vi "CleanUp.vi"(0 "object in":refnum<class "AD2andExtAWG.lvclass">, 5 "error in (no error)":errorcluster) -> (14 "object out":refnum<class "AD2andExtAWG.lvclass">, 19 "error out":errorcluster)   [LabVIEW 2019, in "AD2andExtAWG.lvclass"]
uses:
  AD2andExtAWG.lvclass
  AD2_SDK_class/AD2_SDK.lvclass
  AFG3022B_class/AFG3022B.lvclass
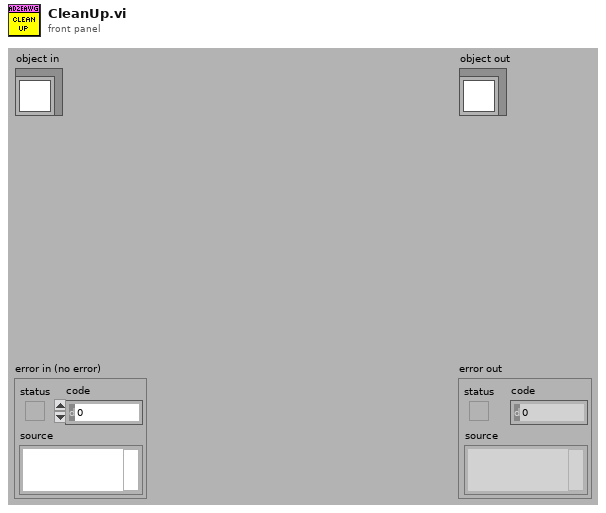
[diagram p1: front panel]
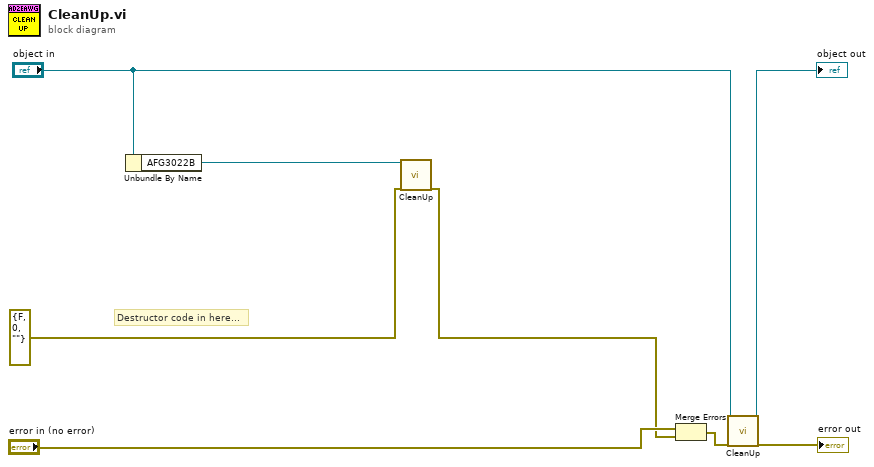
[diagram p0: block diagram]
diagram:
  # "Destructor code in here..."
  n1 = Unbundle By Name("object in") -> ("AFG3022B"=w3:refnum<class "AFG3022B.lvclass">)
  n2 = call-dynamic "CleanUp.vi"("object in"=w3, "error in (no error)"=errorcluster {"status"=FALSE, "code"=0, "source"=""}) -> ("error out"=w1:errorcluster)  [unwired: 16 in, 1 out]
  n3 = Merge Errors("error in (no error)", w1) -> (w7:errorcluster)
  n4 = call-parent "CleanUp.vi"("object in"="object in", "error in (no error)"=w7) -> ("object out"=→"object out":refnum<class "AD2andExtAWG.lvclass">, "error out"=→"error out":errorcluster)  [unwired: 16 in]
